vi "1D Path Array_DeleteEmptyCells.vi"(2 "1D Path Array.IN":path[](array[path])=[path "", path ""]) -> (6 "1D Path Array.OUT":path[](array[path]))   [LabVIEW 2024]
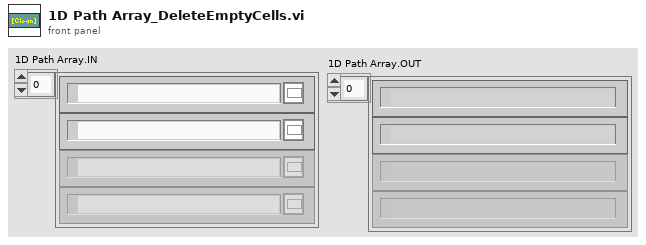
[diagram p1: front panel]
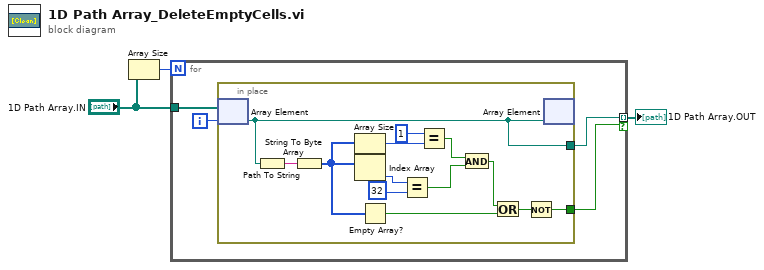
[diagram p0: block diagram]
diagram:
  n1 = Array Size(array="1D Path Array.IN") -> (size(s)=w3:i32)
  n2 = for {
    N: w3 -> [_]
    tunnel: "1D Path Array.IN" -> [w6]
    tunnel: [w4] -> w1 mode=indexing if=w7
    i -> [w5]
    n3 = in-place {
      in-place-border: [w10] -> w7
      in-place-border: [w8] -> w4
      n4 = in-place-array #1(w6, w5) -> (w8:path)
      n5 = Path To String(path=w8) -> (string=w9:string)
      n6 = String To Byte Array(string=w9) -> (unsigned byte array=w18:u8[])
      n7 = Array Size(array=w18) -> (size(s)=w17:i32)
      n8 = Index Array(array=w18) -> (element=w20:u8)  [unwired: 1 in]
      n9 = Empty Array?(array=w18) -> (empty?=w12:bool)
      n10 = Equal?(x=w20, y=u8 32) -> (x = y?=w14:bool)
      n11 = Equal?(x=1, y=w17) -> (x = y?=w15:bool)
      n12 = And(x=w15, y=w14) -> (x .and. y?=w13:bool)
      n13 = Or(x=w13, y=w12) -> (x .or. y?=w11:bool)
      n14 = Not(x=w11) -> (.not. x?=w10:bool)
      n15 = in-place-array #1(w8) -> ()  [unwired: 2 out]
    }
  }
  "1D Path Array.OUT" <- w1
